vi "File IO - Input Test Name_SubVIs-某型振动实验台测试系统.vi"(8 "Error In":errorcluster) -> (0 "Error Out":errorcluster, 2 "OK":bool, 3 "Test Information":cluster{"Test Name":string, "Tester":string}, 4 "测试条件":T1, 5 "粉尘特性":T2)   [LabVIEW 2011]
panel:
  in  "test info":string[][](table)
  in  "Cancel":bool
  in  "Test Information":cluster{"试验名称":string, "试验人":string}
  in  "OK":bool
  # "试验信息"
  # "测试条件"
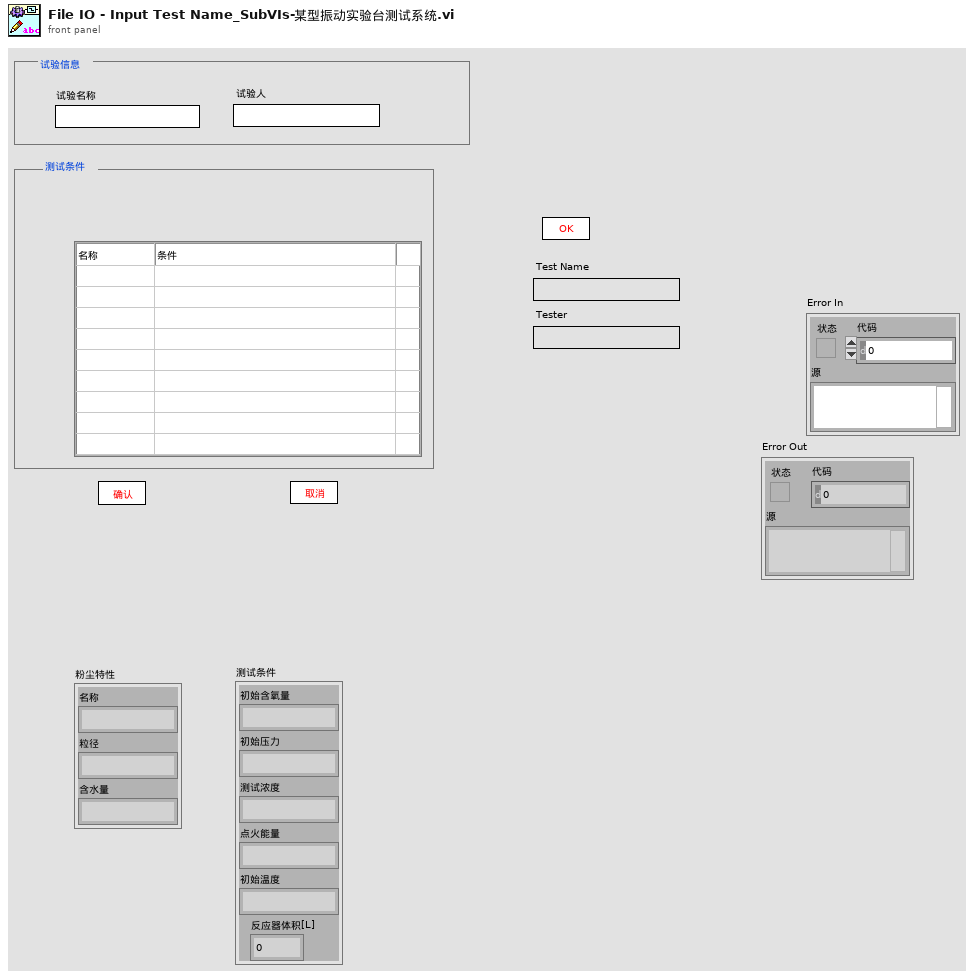
[diagram p1: front panel]
types:
  T1 = typedef "测试条件.ctl" = cluster{"初始含氧量":string, "初始压力":string, "测试浓度":string, "点火能量":string, "初始温度":string, "反应器体积[L]":dbl}
  T2 = typedef "粉尘特性.ctl" = cluster{"名称":string, "粒径":string, "含水量":string}
  T3 = cluster{"初始含氧量":string, "初始压力":string, "测试浓度":string, "点火能量":string, "初始温度":string, "反应器体积[L]":dbl}
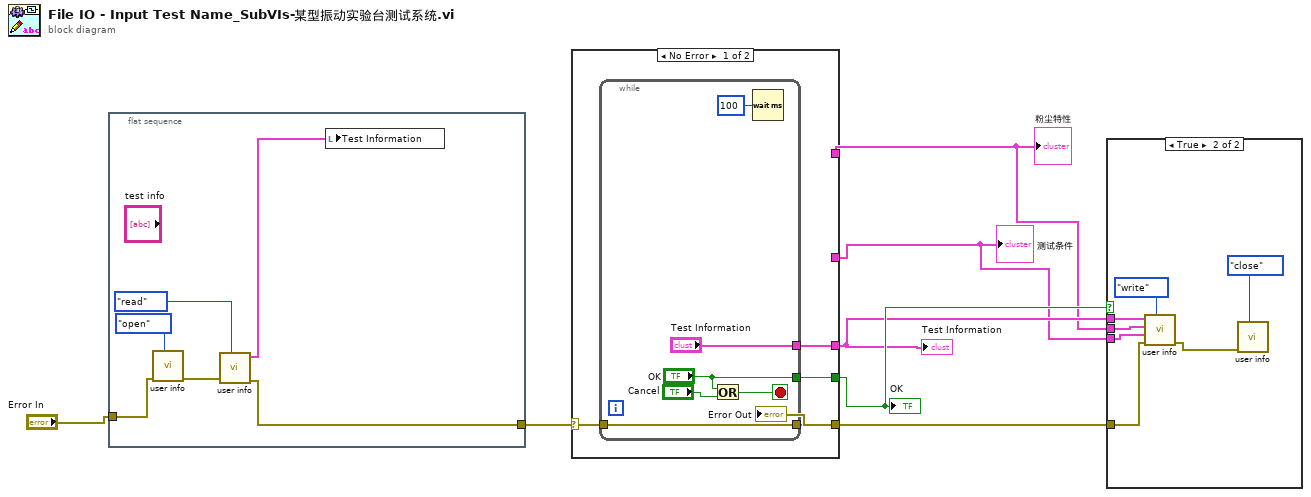
[diagram p0: block diagram]
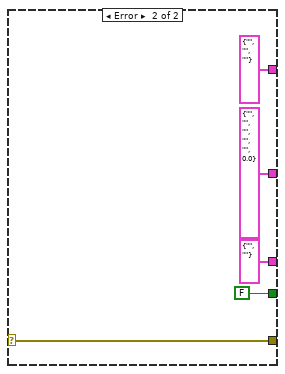
[diagram p3: hidden frame]
diagram:
  n1 = flat-sequence {
    tunnel: "Error In" -> [w9]
    tunnel: [w8] -> w6
    frame #0 {
      n2 = call "user info.vi"("枚举"=enum16{"open", "write", "read", "close"}."open", "error in"=w9) -> ("error out"=w11:errorcluster)  [unwired: 3 in, 6 out]
      n3 = call "user info.vi"("枚举"=enum16{"open", "write", "read", "close"}."read", "error in"=w11) -> ("error out"=w8:errorcluster, "Test Information"=w10:cluster{"Test Name":string, "Tester":string})  [unwired: 3 in, 5 out]
      n4 = local write "Test Information"(w10) -> ()
    }
  }
  n5 = case shown="No Error" w6 {
    selector: w6 -> [w17 w28]
    tunnel: [w16 w28] -> w1
    tunnel: [w15 cluster{"Test Name":string, "Tester":string} {"Test Name"="", "Tester"=""} ("Test Information")] -> w4
    tunnel: [w14 FALSE ("OK")] -> w5
    tunnel: [_ T3 {"初始含氧量"="", "初始压力"="", "测试浓度"="", "点火能量"="", "初始温度"="", "反应器体积[L]"=0.0}] -> w2
    tunnel: [_ cluster{"名称":string, "粒径":string, "含水量":string} {"名称"="", "粒径"="", "含水量"=""}] -> w3
    frame No Error {
      n6 = while {
        tunnel: [w22] -> w16
        tunnel: w17 -> [w22]
        tunnel: ["Test Information"] -> w15
        tunnel: ["OK"] -> w14
        stop <- w19 stop-if-true
        n7 = Or(x="OK", y="Cancel") -> (x .or. y?=w19:bool)
        n8 = Wait (ms)(milliseconds to wait=u32 100 ("等待时间（毫秒）")) -> ()  [unwired: 1 out]
      }
    }
    frame Error {
    }
  }
  "Error Out" <- w1
  "Test Information" <- w4
  "OK" <- w5
  "粉尘特性" <- w3
  "测试条件" <- w2
  n9 = case shown="True" w5 {
    tunnel: w4 -> [_ w33]
    tunnel: w3 -> [_ w32]
    tunnel: w2 -> [_ w31]
    tunnel: w1 -> [_ w29]
    frame False {
    }
    frame True {
      n10 = call "user info.vi"("枚举"=enum16{"open", "write", "read", "close"}."write", "error in"=w29, "测试条件 in"=w31, "粉尘特性 in"=w32, "Test Information in"=w33) -> ("error out"=w30:errorcluster)  [unwired: 6 out]
      n11 = call "user info.vi"("枚举"=enum16{"open", "write", "read", "close"}."close", "error in"=w30) -> ()  [unwired: 3 in, 7 out]
    }
  }
